vi "Draw.vi"(7 "Stimulus Snippet":T1, 8 "error in (no error)":errorcluster, 9 "StimulusImageIn":T2, 10 "CalibrationImage":T2, 11 "JustHeadEllipseRatioRails in":refnum<class "JustHeadEllipseRatioRails.lvclass">) -> (0 "error out":errorcluster, 1 "StimulusImageOut":T2, 3 "JustHeadEllipseRatioRails out":refnum<class "JustHeadEllipseRatioRails.lvclass">)   [LabVIEW 2019, in "JustHeadEllipseRatioRails.lvclass"]
uses:
  JustHeadEllipseRatioRails.lvclass
  <vilib>/vision/Image Controls.llb/IMAQ Image.ctl
  StimulusSnippetCluster.ctl
  JustHeadEllipseRatioRails.lvclass/JustHeadEllipseRatioRails.ctl
  ParametersGlobal.vi
  <vilib>/vision/NI_Vision_Development_Module.lvlib
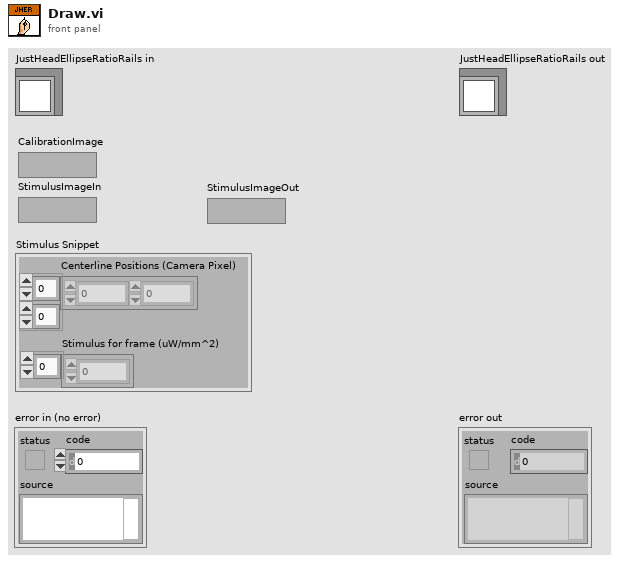
[diagram p1: front panel]
types:
  T1 = typedef "StimulusSnippetCluster.ctl" = cluster{"Centerline Positions (Camera Pixel)":sgl[][], "Stimulus for frame (uW/mm^2)":sgl[]}
  T2 = typedef "IMAQ Image.ctl" = refnum<image>
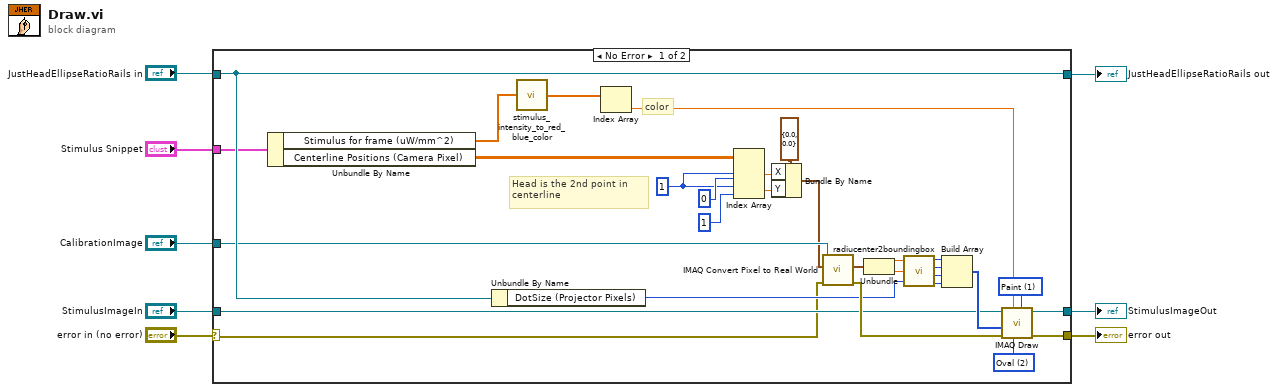
[diagram p0: block diagram]
diagram:
  n1 = case shown="No Error" "error in (no error)" {
    selector: "error in (no error)" -> [w19 w41]
    tunnel: [w12 w41] -> w1
    tunnel: [w20 w40] -> w3
    tunnel: "JustHeadEllipseRatioRails in" -> [w20 w40]
    tunnel: [w13 w39] -> w2
    tunnel: "StimulusImageIn" -> [w26 w39]
    tunnel: "Stimulus Snippet" -> [w17 _]
    tunnel: "CalibrationImage" -> [w16 _]
    frame No Error {
      w9 = 1 ("index (row)")
      w11 = u16 1 items=["Frame", "Paint", "Invert Frame", "Invert Paint"] ("Draw Mode")
      w38 = u16 2 items=["Line", "Rectangle", "Oval"] ("Shape to draw")
      # "Head is the 2nd point in centerline"
      # "color"
      n2 = Unbundle By Name(w17) -> ("Stimulus for frame (uW/mm^2)"=w18:sgl[], "Centerline Positions (Camera Pixel)"=w10:sgl[][])
      n3 = Unbundle By Name(w20) -> ("DotSize (Projector Pixels)"=w21:i32)
      n4 = call "stimulus_intensity_to_red_blue_color.vi"("StimulusIntensityForFrame"=w18) -> ("StimulusColorForFrame"=w22:sgl[])
      n5 = Index Array(array=w22) -> (element=w15:sgl)  [unwired: 1 in]
      n6 = Index Array(array=w10, index (row) #1=w9, index (col) #1=0 ("disabled index (col)"), index (row) #2=w9, index (col) #2=1 ("disabled index (col)")) -> (element #1=w24:sgl, element #2=w23:sgl)
      n7 = Bundle By Name(cluster=cluster{"X":sgl, "Y":sgl} {"X"=0.0, "Y"=0.0} ("Camera Point"), "X"=w24, "Y"=w23) -> (w14:cluster{"X":sgl, "Y":sgl})
      n8 = call "IMAQ Convert Pixel to Real World"("error in (no error)"=w19, "Pixel Coordinates"=w14, "Calibrated Image"=w16) -> ("error out"=w29:errorcluster, "Real World Coordinates"=w30:cluster{"X":sgl, "Y":sgl})  [unwired: 3 in, 4 out]
      n9 = Unbundle(w30) -> ("X"=w32:sgl, "Y"=w31:sgl)
      n10 = call "radiucenter2boundingbox.vi"("Radius"=w21, "ycenter"=w31, "xcenter"=w32) -> ("Bottom"=w33:i32, "Right"=w34:i32, "Top"=w35:i32, "Left"=w36:i32)  [unwired: 2 in]
      n11 = Build Array(w36, w35, w34, w33) -> (w37:i32[])
      n12 = call "IMAQ Draw"("Draw Mode"=w11, "Shape to draw"=w38, "Pixel Color"=w15, "error in (no error)"=w29, "Coordinates"=w37, "Image Src"=w26) -> ("error out"=w12:errorcluster, "Image Dst Out"=w13:T2)  [unwired: 4 in]
    }
    frame Error {
    }
  }
  "error out" <- w1
  "JustHeadEllipseRatioRails out" <- w3
  "StimulusImageOut" <- w2
